vi "Door Open.vi"(10 "Infeed Door In Auto":bool, 11 "Infeed Door In":bool) -> (3 "Infeed Door Out":bool)   [LabVIEW 2014]
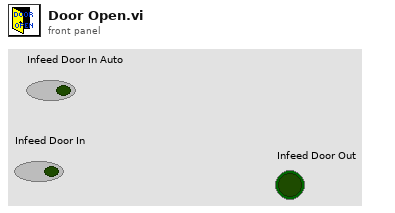
[diagram p1: front panel]
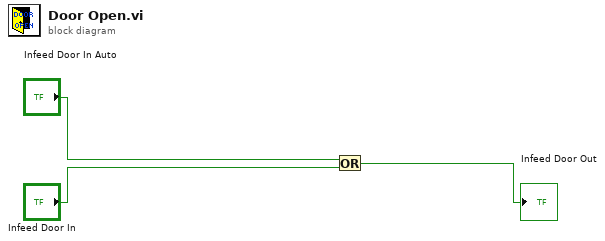
[diagram p0: block diagram]
diagram:
  n1 = Or(x="Infeed Door In Auto", y="Infeed Door In") -> (x .or. y?=→"Infeed Door Out":bool)
